vi "Model - DeInit.vi"(8 "error in (no error)":errorcluster, 11 "View Model":T1) -> (0 "error out":errorcluster)   [LabVIEW 2017]
doc: "De-Initialize all ueser events and DVRs of View Model."
uses:
  Controls/View Model.ctl
  Error Handler/Controls/Error Model.ctl
  Error Handler/Controls/Error Data.ctl
  Error Handler/Controls/Error Type.ctl
  Controls/Shared Model.ctl
  Configuration/Controls/Config Model.ctl
  Configuration/Controls/Config CMD.ctl
  Configuration/Controls/Config Data.ctl
  ATM Controller/Controls/Controller Model.ctl
  ATM Controller/Controls/Controller Overhead.ctl
  ATM Controller/Controls/Controller States.ctl
  ATM Controller/Controls/Controller Message Data.ctl
  ATM Controller/Controls/Controller Message Name.ctl
  ATM Controller/Controls/Controller CMD.ctl
  Views/User Console View/Controls/User Console - Transaction Enum.ctl
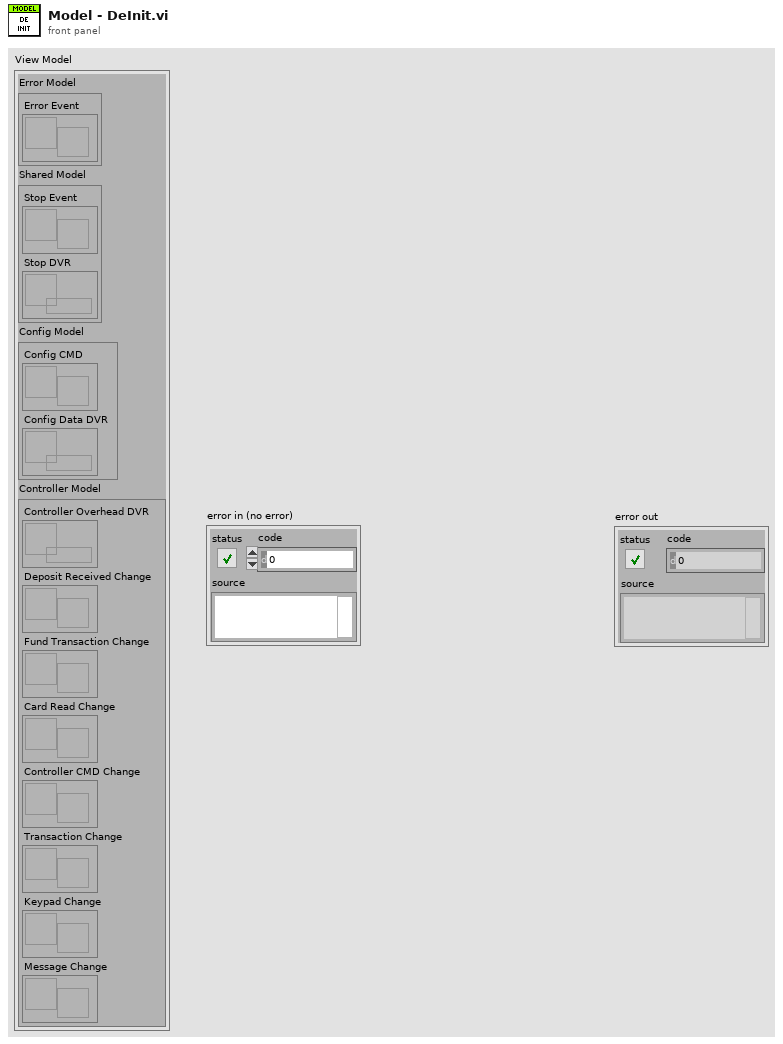
[diagram p1: front panel]
types:
  T1 = typedef "View Model.ctl" = cluster{"Error Model":T2, "Shared Model":T3, "Config Model":T4, "Controller Model":T5}
  T2 = typedef "Error Model.ctl" = cluster{"Error Event":refnum<user-event>}
  T3 = typedef "Shared Model.ctl" = cluster{"Stop Event":refnum<user-event>, "Stop DVR":refnum<data-value>}
  T4 = typedef "Config Model.ctl" = cluster{"Config CMD":refnum<user-event>, "Config Data DVR":refnum<data-value>}
  T5 = typedef "Controller Model.ctl" = cluster{"Controller Overhead DVR":refnum<data-value>, "Deposit Received Change":refnum<user-event>, "Fund Transaction Change":refnum<user-event>, "Card Read Change":refnum<user-event>, "Controller CMD Change":refnum<user-event>, "Transaction Change":refnum<user-event>, "Keypad Change":refnum<user-event>, "Message Change":refnum<user-event>}
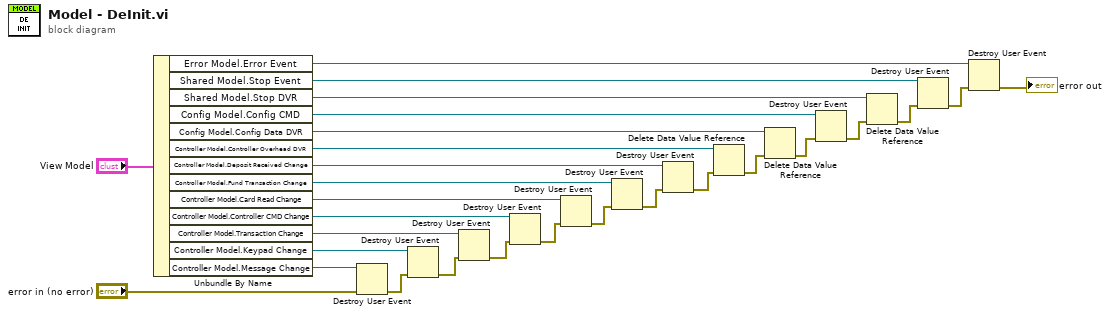
[diagram p0: block diagram]
diagram:
  n1 = Unbundle By Name("View Model") -> ("Error Model.Error Event"=w4:refnum<user-event>, "Shared Model.Stop Event"=w6:refnum<user-event>, "Shared Model.Stop DVR"=w8:refnum<data-value>, "Config Model.Config CMD"=w10:refnum<user-event>, "Config Model.Config Data DVR"=w12:refnum<data-value>, "Controller Model.Controller Overhead DVR"=w14:refnum<data-value>, "Controller Model.Deposit Received Change"=w16:refnum<user-event>, "Controller Model.Fund Transaction Change"=w18:refnum<user-event>, "Controller Model.Card Read Change"=w20:refnum<user-event>, "Controller Model.Controller CMD Change"=w22:refnum<user-event>, "Controller Model.Transaction Change"=w24:refnum<user-event>, "Controller Model.Keypad Change"=w26:refnum<user-event>, "Controller Model.Message Change"=w27:refnum<user-event>)
  n2 = Destroy User Event(user event=w27, error in="error in (no error)") -> (error out=w25:errorcluster)
  n3 = Destroy User Event(user event=w26, error in=w25) -> (error out=w23:errorcluster)
  n4 = Destroy User Event(user event=w24, error in=w23) -> (error out=w21:errorcluster)
  n5 = Destroy User Event(user event=w22, error in=w21) -> (error out=w19:errorcluster)
  n6 = Destroy User Event(user event=w20, error in=w19) -> (error out=w17:errorcluster)
  n7 = Destroy User Event(user event=w18, error in=w17) -> (error out=w15:errorcluster)
  n8 = Destroy User Event(user event=w16, error in=w15) -> (error out=w13:errorcluster)
  n9 = Delete Data Value Reference(data value reference=w14, error in=w13) -> (error out=w11:errorcluster)  [unwired: 1 out]
  n10 = Delete Data Value Reference(data value reference=w12, error in=w11) -> (error out=w9:errorcluster)  [unwired: 1 out]
  n11 = Destroy User Event(user event=w10, error in=w9) -> (error out=w7:errorcluster)
  n12 = Delete Data Value Reference(data value reference=w8, error in=w7) -> (error out=w5:errorcluster)  [unwired: 1 out]
  n13 = Destroy User Event(user event=w6, error in=w5) -> (error out=w3:errorcluster)
  n14 = Destroy User Event(user event=w4, error in=w3) -> (error out=→"error out":errorcluster)
